vi "ScaledWaveform-AddResultChannel.vi"(8 "Error in":errorcluster, 11 "Custom Device ref":T1 format="%.0x") -> (0 "Error out":errorcluster, 3 "Custom Device ref out":T1 format="%.0x")   [LabVIEW 2015, in "Waveform-Processing-Custom-Device Shared.lvlib" / "Scaled Waveform.lvlib"]
uses:
  Scaled Waveform.lvlib
  <vilib>/NI Veristand/Custom Device API/Custom Device Item Ref.ctl
  <vilib>/NI Veristand/Custom Device API/Custom Device Waveform.ctl
  <vilib>/NI Veristand/Custom Device API/Custom Device Waveform DataType.ctl
  NationalInstruments.VeriStand.SystemStorage
  Constants.vi
  <vilib>/NI Veristand/Custom Device API/Get Item Property (Dependent Node Pointer).vi
  <vilib>/NI Veristand/Custom Device API/Set Item Property (Dependent Node Pointer).vi
  <vilib>/NI VeriStand/Custom Device API/Custom Device API.lvlib
  Waveform-Processing-Custom-Device Shared.lvlib
  System Explorer/Waveform-Processing-Custom-Device System Explorer.lvlib
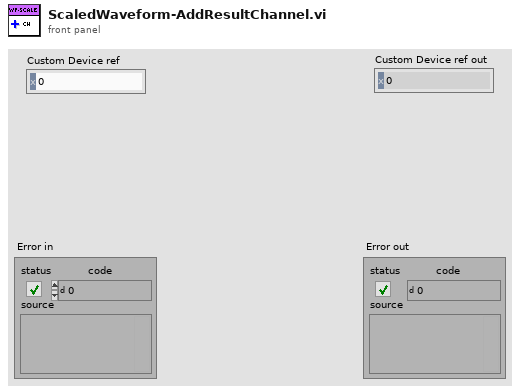
[diagram p1: front panel]
types:
  T1 = typedef "Custom Device API.lvlib/Custom Device Item Ref.ctl" = u64
  T2 = typedef "Custom Device API.lvlib/Custom Device Waveform.ctl" = cluster{"Data Type":T3, "Units":string}
  T3 = typedef "Custom Device API.lvlib/Custom Device Waveform DataType.ctl" = enum16{"Double", "Complex Double"}
  T4 = typedef "Custom Device API.lvlib/Custom Device Pointer.ctl" = refnum<k24>
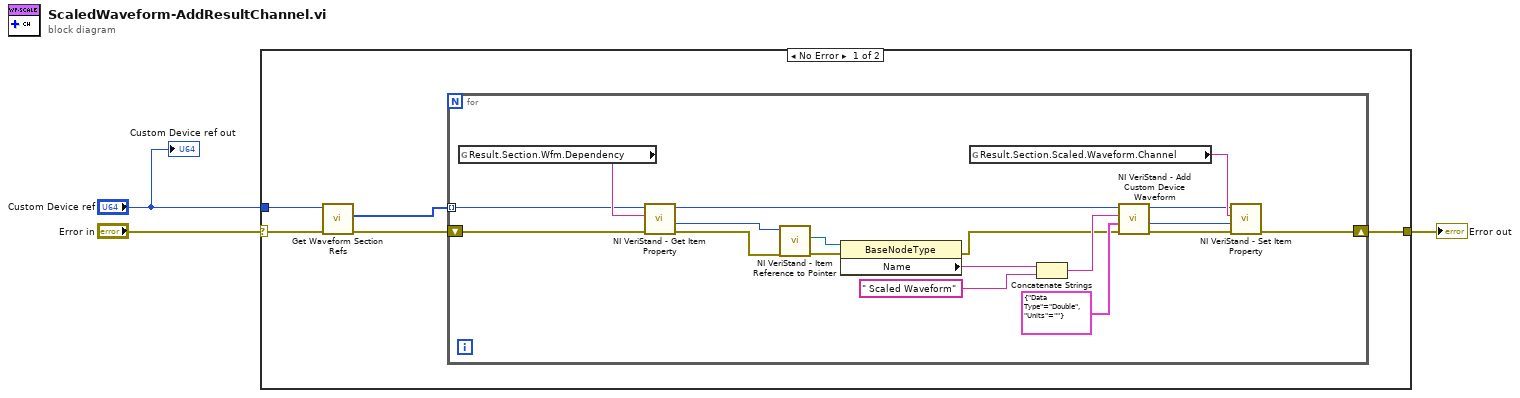
[diagram p0: block diagram]
diagram:
  n1 = case shown="No Error" "Error in" {
    selector: "Error in" -> [w8 w27]
    tunnel: "Custom Device ref" -> [w7 _]
    tunnel: [w4 w27] -> w2
    frame No Error {
      n2 = call "Get Waveform Section Refs.vi"("Error in"=w8, "Device Ref in"=w7) -> ("Error out"=w6:errorcluster, "Result Section Refs"=w5:T1[])  [unwired: 7 in, 1 out]
      n3 = for {
        tunnel: w5 -> [w20] mode=indexing
        shift-right: [w14] -> w4
        shift-left: w6 -> [w19]
        n4 = global read "Constants.vi" "Result.Section.Wfm.Dependency"() -> (w26:string)
        n5 = call-poly <vilib>:"NI VeriStand - Get Item Property.vi"("error in (no error)"=w19, "Property Name"=w26, "Item Ref in"=w20) -> ("error out"=w23:errorcluster, "Dependent Node Ref"=w24:T1, "Item Ref out"=w11:T1)  [unwired: 5 in, 1 out]
        n6 = call <vilib>:"NI VeriStand - Item Reference to Pointer.vi"("error in (no error)"=w23, "Item Ref in"=w24) -> ("error out"=w22:errorcluster, "Node Pointer"=w12:T4)  [unwired: 6 in, 2 out]
        n7 = property class="BaseNodeType"(reference=w12, error in=w22) -> (error out=w15:errorcluster, "Name"=w16:string)  [unwired: 1 out]
        n8 = global read "Constants.vi" "Result.Section.Scaled.Waveform.Channel"() -> (w18:string)
        n9 = Concatenate Strings(w16, " Scaled Waveform" ("Property Name")) -> (w25:string)
        n10 = call <vilib>:"NI VeriStand - Add Custom Device Waveform.vi"("error in (no error)"=w15, "Waveform"=T2 {"Data Type"=enum."Double", "Units"=""}, "Waveform Name"=w25, "Parent Ref in"=w11) -> ("error out"=w13:errorcluster, "Waveform Ref"=w9:T1, "Parent Ref out"=w10:T1)  [unwired: 4 in, 1 out]
        n11 = call-poly <vilib>:"NI VeriStand - Set Item Property.vi"("error in (no error)"=w13, "Dependent Node Ref"=w9, "Property Name"=w18, "Item Ref in"=w10) -> ("error out"=w14:errorcluster)  [unwired: 5 in, 2 out]
      }
    }
    frame Error {
    }
  }
  "Error out" <- w2
  "Custom Device ref out" <- "Custom Device ref"
